vi "Find innermost loop.vi"(1 "Script":string="stuff\nloop(3){repeat1\nloop(2){repeat2}}") -> (0 "No nested loops?":bool, 2 "Offset of inner loop start":i32=12, 3 "Offset of inner loop end":i32=-1, 4 "Any more loops?":bool, 5 "Script before inner loop":string, 6 "Inner loop":string, 7 "Script after inner loop":string)   [LabVIEW 2019]
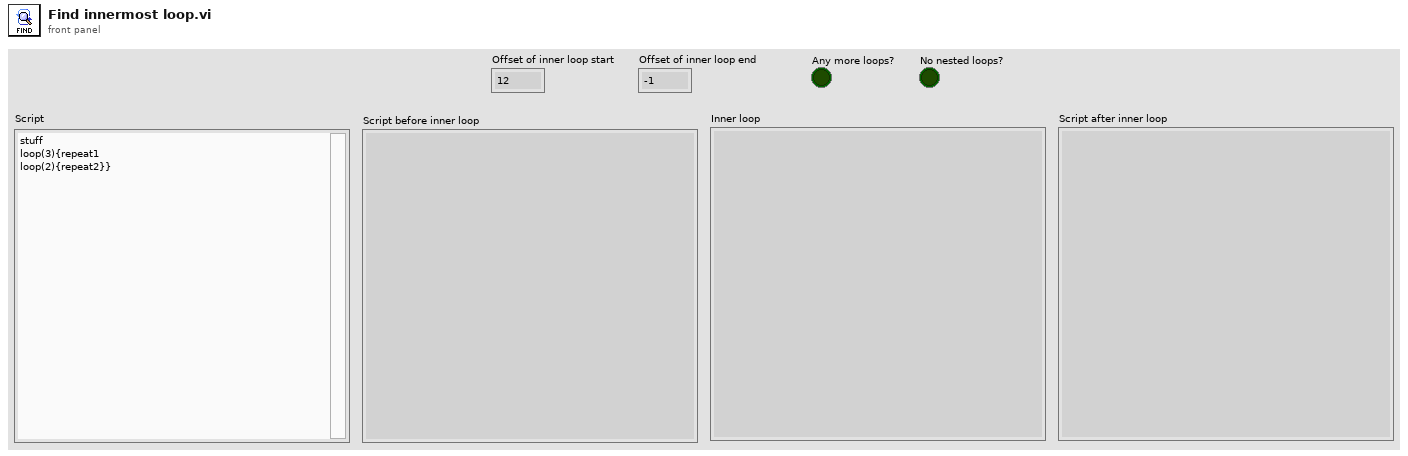
[diagram p1: front panel]
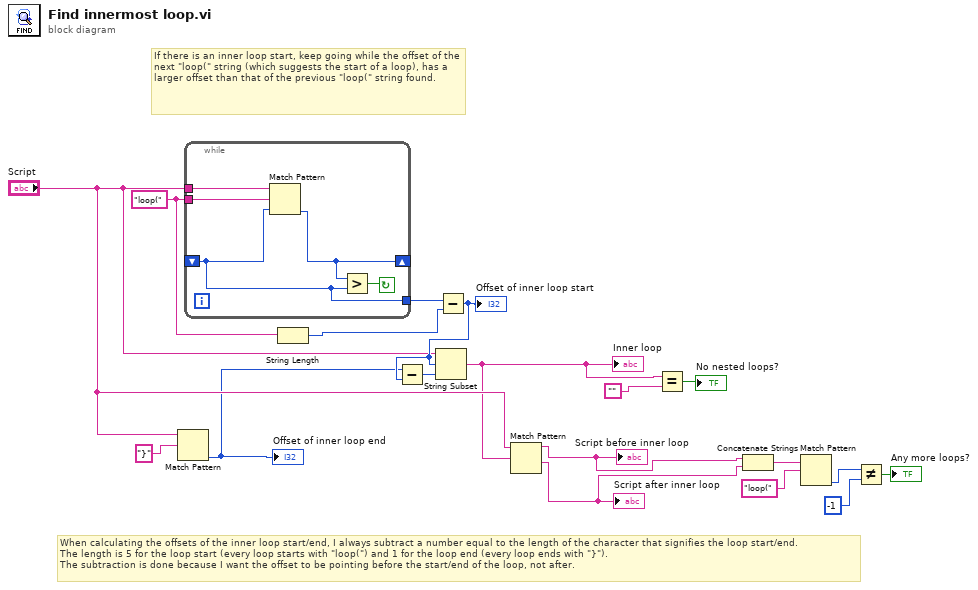
[diagram p0: block diagram]
diagram:
  w17 = "loop(" ("regular expression")
  # "When calculating the offsets of the inner loop start/end, I always subtract a number equal to the length of the character that signifies the loop start/end.\nThe length is 5 for the loop start (every loop starts with \"loop(\") and 1 for the loop end (every loop ends with \"}\").\nThe subtraction is done because I want the offset to be pointing before the start/end of the loop, not after."
  # "If there is an inner loop start, keep going while the offset of the next \"loop(\" string (which suggests the start of a loop), has a larger offset than that of the previous \"loop(\" string found."
  n1 = Match Pattern(string="Script", regular expression="}") -> (offset past match=w11:i32)  [unwired: 1 in, 3 out]
  "Offset of inner loop end" <- w11
  n2 = while {
    tunnel: "Script" -> [w23]
    shift-right: [w22] -> _
    shift-left: _ -> [w20]
    tunnel: [w20] -> w15
    tunnel: w17 -> [w19]
    stop <- w21 continue-if-true
    n3 = Match Pattern(string=w23, regular expression=w19, offset (0)=w20) -> (offset past match=w22:i32)  [unwired: 3 out]
    n4 = Greater?(x=w22, y=w20) -> (0:w21:bool)
  }
  n5 = String Length(string=w17) -> (length=w16:i32)
  n6 = Subtract(x=w15, y=w16) -> (x-y=w14:i32)
  "Offset of inner loop start" <- w14
  n7 = Subtract(x=w11, y=w14) -> (x-y=w18:i32)
  n8 = String Subset(string="Script", offset (0)=w14, length (rest)=w18) -> (substring=w2:string)
  "Inner loop" <- w2
  n9 = Match Pattern(string="Script", regular expression=w2) -> (before substring=w10:string, after substring=w9:string)  [unwired: 1 in, 2 out]
  "Script before inner loop" <- w10
  "Script after inner loop" <- w9
  n10 = Equal?(x=w2, y="") -> (x = y?=→"No nested loops?":bool)
  n11 = Concatenate Strings(w10, w9) -> (w8:string)
  n12 = Match Pattern(string=w8, regular expression="loop(") -> (offset past match=w5:i32)  [unwired: 1 in, 3 out]
  n13 = Not Equal?(x=w5, y=-1) -> (x != y?=→"Any more loops?":bool)
